vi "IO_create_frequency_array.vi"(9 "cor":T1) -> (1 "Array 2":string[](array[string]), 2 "Array":dbl[](array[numeric]))   [LabVIEW 2012]
doc: "Creates an array of frequency values corresponding to an input spectrum. Each element in the frequency for each data value in the spectra."
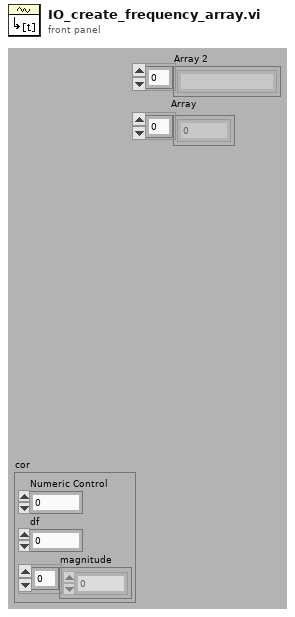
[diagram p1: front panel]
types:
  T1 = cluster{"Numeric Control":dbl, "df":dbl, "magnitude":dbl[]}
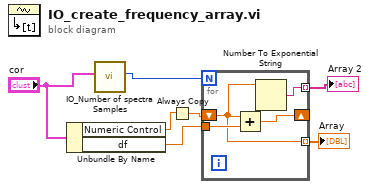
[diagram p0: block diagram]
diagram:
  n1 = Unbundle By Name("cor") -> ("Numeric Control"=w5:dbl, "df"=w6:dbl)
  n2 = call "IO_Number of spectra Samples.vi"("cor"="cor") -> ("number of samples"=w3:i32)  [unwired: 10 in]
  n3 = Always Copy(1:w5) -> (0:w7:dbl)
  n4 = for {
    N: w3 -> [_]
    shift-right: [w10] -> _
    shift-left: w7 -> [w8]
    tunnel: w6 -> [w11]
    tunnel: [w9] -> w2 mode=indexing
    tunnel: [w8] -> w1 mode=indexing
    n5 = Add(x=w8, y=w11) -> (x+y=w10:dbl)
    n6 = Number To Exponential String(number=w8) -> (E-format string=w9:string)  [unwired: 3 in]
  }
  "Array 2" <- w2
  "Array" <- w1
